vi "GetDPAFromSRIM.vi"(10 "Start Index":i32, 11 "Tab Array":string[][](array[string])) -> (3 "DPA":dbl)   [LabVIEW 2012]
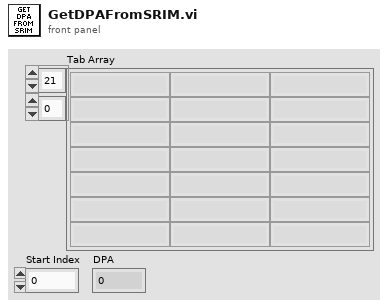
[diagram p1: front panel]
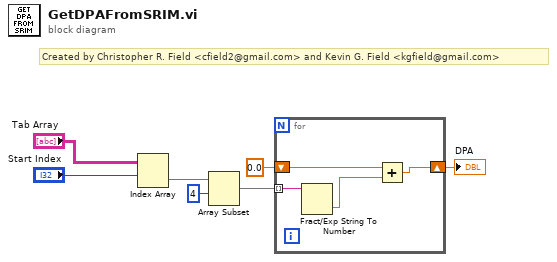
[diagram p0: block diagram]
diagram:
  # "Created by Christopher R. Field <cfield2@gmail.com> and Kevin G. Field <kgfield@gmail.com>"
  n1 = Index Array(array="Tab Array", index (row)="Start Index") -> (element=w5:string[])  [unwired: 1 in]
  n2 = Array Subset(array=w5, index=4) -> (w3:string[])  [unwired: 1 in]
  n3 = for {
    tunnel: w3 -> [w11] mode=indexing
    shift-right: [w8] -> w1
    shift-left: 0.0 -> [w9]
    n4 = Fract/Exp String To Number(string=w11) -> (number=w10:dbl)  [unwired: 3 in, 1 out]
    n5 = Add(x=w9, y=w10) -> (x+y=w8:dbl)
  }
  "DPA" <- w1
